vi "Turret.vi"() -> ()   [LabVIEW 2019]
uses:
  SubVI/Time Global.vi
  Turret Global.vi
  <vilib>/addons/control/pid/pid.llb/PID (DBL).vi
  <vilib>/addons/control/pid/NI_PID_pid.lvlib
panel:
  in  "Position Factor (1)":dbl=4.08666 format="%#_13g"
  in  "y":dbl=0.8
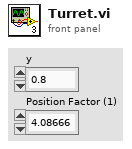
[diagram p1: front panel]
types:
  T1 = typedef "WPI_MotorControlDeviceRef.ctl" = cluster{"DeviceStatus":errorcluster, "Type":T2, "PWM":cluster{"PWM Channel":T3, "DeadBand":T4}, "CAN":cluster{"Device Number":u8, "SetOutput VI Ref":variant, "GetOutput VI Ref":variant, "Enable VI Ref":variant, "Disable VI Ref":variant, "Data":variant}, "Invert":bool, "DIO PWM":cluster{"PWM \"Enable\" Channel":T3, "DIOChannel":T5, "PWM Rate":dbl}}
  T2 = typedef "WPI_MotorControlType.ctl" = enum16{"PWM", "CAN", "DIO PWM"}
  T3 = typedef "FPGA_DIOPWMChannel.ctl" = enum8{"PWM 0", "PWM 1", "PWM 2", "PWM 3", "PWM 4", "PWM 5", "PWM 6", "PWM 7", "PWM 8", "PWM 9", "PWM MXP 0", "PWM MXP 1", "PWM MXP 2", "PWM MXP 3", "PWM MXP 4", "PWM MXP 5", "PWM MXP 6", "PWM MXP 7", "PWM MXP 8", "PWM MXP 9", "Invalid"}
  T4 = typedef "WPI_PWMDeadband.ctl" = cluster{"Name":string, "maxPositivePwm":i32, "minPositivePwm":i32, "centerPwm":i32, "maxNegativePwm":i32, "minNegativePwm":i32, "angularRange":u16}
  T5 = typedef "FPGA_DIOChannel.ctl" = enum8{"DIO 0", "DIO 1", "DIO 2", "DIO 3", "DIO 4", "DIO 5", "DIO 6", "DIO 7", "DIO 8", "DIO 9", "DIO MXP 0", "DIO MXP 1", "DIO MXP 2", "DIO MXP 3", "DIO MXP 4", "DIO MXP 5", "DIO MXP 6", "DIO MXP 7", "DIO MXP 8", "DIO MXP 9", "DIO MXP 10", "DIO MXP 11", "DIO MXP 12", "DIO MXP 13", "DIO MXP 14", "DIO MXP 15", "SPI Port CS1", "SPI Port CS2", "SPI Port CS3", "SPI Port MISO", "SPI Port MOSI", "Invalid"}
  T6 = cluster{"proportional gain (Kc)":dbl, "integral time (Ti, min)":dbl, "derivative time (Td, min)":dbl}
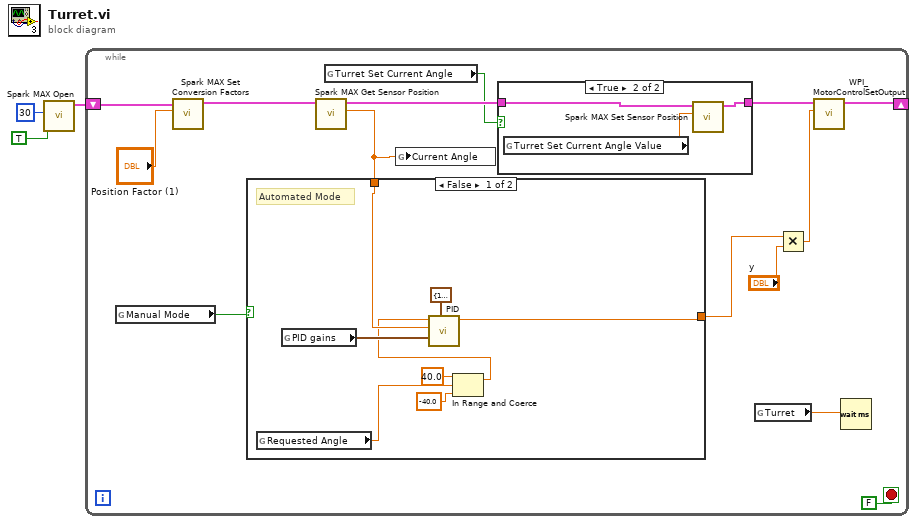
[diagram p0: block diagram]
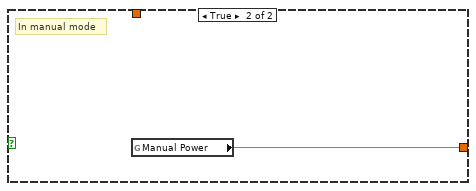
[diagram p3: hidden frame]
diagram:
  n1 = call <vilib>:"Spark MAX Open.vi"("Invert"=TRUE, "Device Number"=u8 30) -> ("MotorControlDeviceRef"=w3:T1)  [unwired: 8 in, 1 out]
  n2 = while {
    shift-right: [w14] -> _
    shift-left: w3 -> [w13]
    stop <- FALSE stop-if-true
    n3 = global read "Turret Global.vi" "Manual Mode"() -> (w15:bool)
    n4 = call <vilib>:"Spark MAX Set Conversion Factors.vi"("Position Factor (1)"="Position Factor (1)", "MotorControlDeviceRef in"=w13) -> ("MotorControlDeviceRef out"=w12:T1)  [unwired: 8 in, 1 out]
    n5 = call <vilib>:"Spark MAX Get Sensor Position.vi"("MotorControlDevRef in"=w12) -> ("Sensor Position"=w8:dbl, "MotorControlDevRef out"=w6:T1)  [unwired: 7 in, 2 out]
    n6 = case shown="False" w15 {
      tunnel: [w26 w30] -> w11
      tunnel: w8 -> [w29 _]
      frame False {
        # "Automated Mode"
        n7 = global read "Turret Global.vi" "Requested Angle"() -> (w23:dbl)
        n8 = global read "Turret Global.vi" "PID gains"() -> (w27:T6)
        n9 = In Range and Coerce(upper limit=40.0, x=w23, lower limit=-40.0) -> (coerced(x)=w22:dbl)  [unwired: 1 out]
        n10 = call-poly <vilib>:"PID.vi"("output range"=cluster{"output high":dbl, "output low":dbl} {"output high"=1.0, "output low"=-1.0}, "PID gains"=w27, "process variable"=w29, "setpoint"=w22) -> ("output"=w26:dbl)  [unwired: 6 in, 1 out]
      }
      frame True {
        # "In manual mode"
        n11 = global read "Turret Global.vi" "Manual Power"() -> (w30:dbl)
      }
    }
    n12 = global read "Turret Global.vi" "Turret Set Current Angle"() -> (w4:bool)
    n13 = global write "Turret Global.vi" "Current Angle"(w8) -> ()
    n14 = case shown="True" w4 {
      tunnel: w6 -> [w18 w21]
      tunnel: [w18 w20] -> w5
      frame False {
      }
      frame True {
        n15 = global read "Turret Global.vi" "Turret Set Current Angle Value"() -> (w19:dbl)
        n16 = call <vilib>:"Spark MAX Set Sensor Position.vi"("Position"=w19, "MotorControlDeviceRef"=w21) -> ("MotorControlDeviceRef"=w20:T1)  [unwired: 8 in, 1 out]
      }
    }
    n17 = global read "Time Global.vi" "Turret"() -> (w16:dbl)
    n18 = Multiply(x=w11, y="y") -> (x*y=w10:dbl)
    n19 = call <vilib>:"WPI_MotorControlSetOutput.vi"("Output"=w10, "MotorControlDevRef"=w5) -> ("MotorControlDevRef"=w14:T1)  [unwired: 7 in, 2 out]
    n20 = Wait (ms)(milliseconds to wait=w16) -> ()  [unwired: 1 out]
  }
